vi "plots2DAnd3D.vi"() -> ()   [LabVIEW 2014]
uses:
  <vilib>/Math Plots/2D Math Plots/2D Error Bar/2D Error Bar XCtrl/2D Error Bar.xctl
  <vilib>/Math Plots/3D Math Plots/3D Contour/3D Contour XCtrl/3D Contour.xctl
  <vilib>/Math Plots/2D Math Plots/2D Error Bar/2D Error Bar Datatype/Public/Plot Helper (Percentage).vi
  <vilib>/Math Plots/3D Math Plots/3D Contour/3D Contour Datatype/Public/Plot Helper (Matrix).vi
  <vilib>/Math Plots/2D Math Plots/2D Error Bar/2D Error Bar Datatype/2D Error Bar Datatype.lvclass
  <vilib>/Math Plots/3D Math Plots/3D Contour/3D Contour Datatype/3D Contour Datatype.lvclass
panel:
  out "Contour Plotting Error":errorcluster
  in  "Frequency":dbl(knob) scale=0.0..100.0
  out "3D Contour":refnum<class "3D Plot Datatype.lvclass">[](xcontrol)
  in  "Lower Error (%)":dbl(slide) scale=0.0..10.0
  in  "Upper Error (%)":dbl(slide) scale=0.0..10.0
  out "Errorbar Plotting Error":errorcluster
  in  "Number of Points":i32(knob) scale=0.0..200.0
  out "Error Bar Plot":refnum<class "2D Plot Datatype.lvclass">[](xcontrol) caption="2D Error Bar"
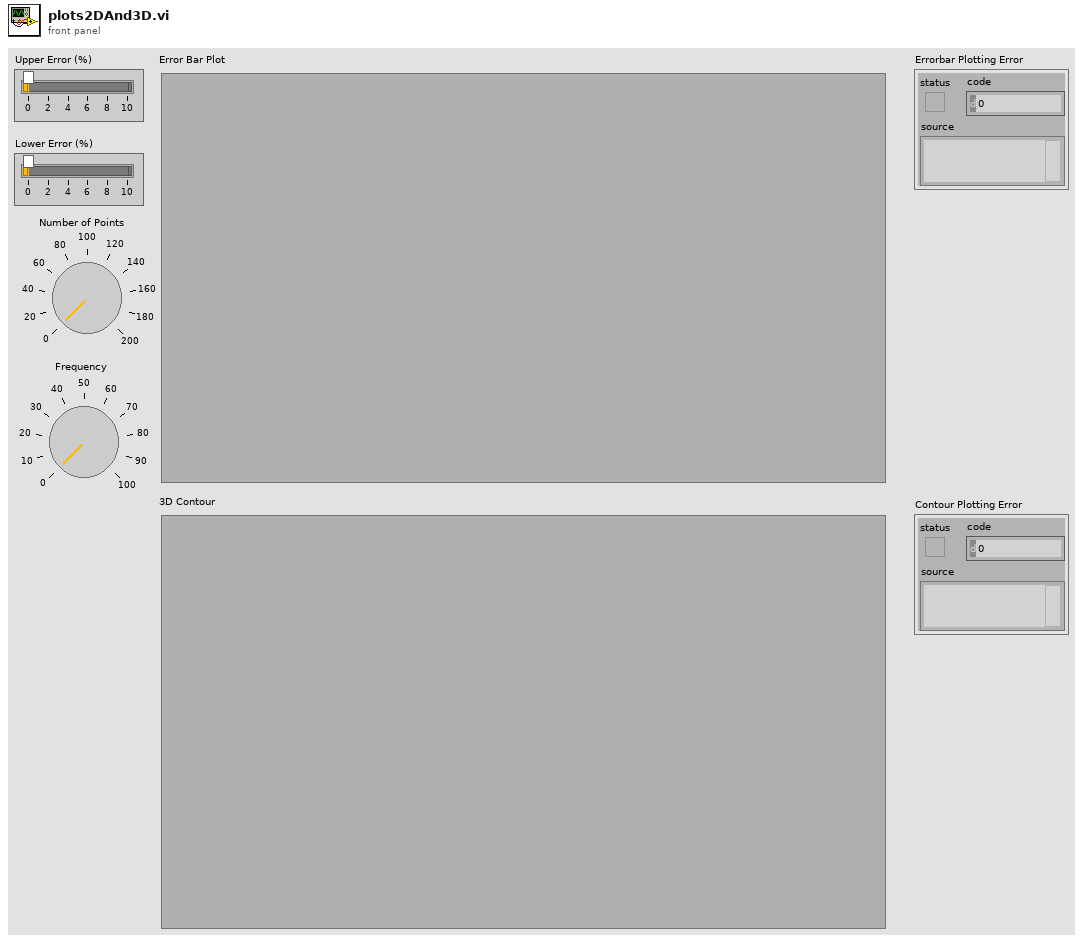
[diagram p1: front panel]
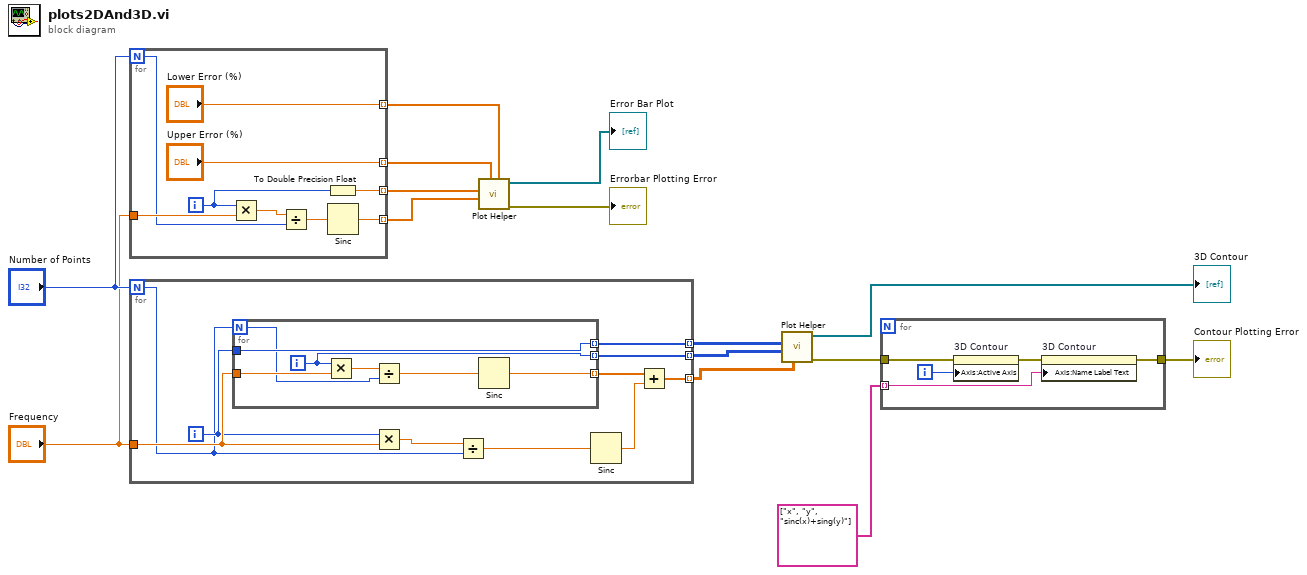
[diagram p0: block diagram]
diagram:
  n1 = for {
    N: "Number of Points" -> [w16]
    tunnel: [w24] -> w14 mode=indexing
    tunnel: [w23] -> w13 mode=indexing
    tunnel: ["Lower Error (%)"] -> w11 mode=indexing
    tunnel: ["Upper Error (%)"] -> w10 mode=indexing
    tunnel: "Frequency" -> [w19]
    i -> [w20]
    n2 = Multiply(x=w20, y=w19) -> (x*y=w17:dbl)
    n3 = Divide(x=w17, y=w16) -> (x/y=w18:dbl)
    n4 = To Double Precision Float(number=w20) -> (double precision float=w23:dbl)
    n5 = Sinc(1:w18) -> (0:w24:dbl)
  }
  n6 = for {
    N: "Number of Points" -> [w25]
    tunnel: [w32] -> w7 mode=indexing
    tunnel: "Frequency" -> [w31]
    tunnel: [w29] -> w5 mode=indexing
    tunnel: [w28] -> w4 mode=indexing
    i -> [w30]
    n7 = for {
      N: w25 -> [w35]
      tunnel: [w41] -> w33 mode=indexing
      tunnel: w31 -> [w39]
      tunnel: [w38] -> w29 mode=indexing
      tunnel: w30 -> [w38]
      tunnel: [w37] -> w28 mode=indexing
      i -> [w37]
      n8 = Multiply(x=w37, y=w39) -> (x*y=w40:dbl)
      n9 = Divide(x=w40, y=w35) -> (x/y=w36:dbl)
      n10 = Sinc(1:w36) -> (0:w41:dbl)
    }
    n11 = Multiply(x=w30, y=w31) -> (x*y=w27:dbl)
    n12 = Divide(x=w27, y=w25) -> (x/y=w26:dbl)
    n13 = Sinc(1:w26) -> (0:w34:dbl)
    n14 = Add(x=w33, y=w34) -> (x+y=w32:dbl[])
  }
  n15 = call-poly <vilib>:"Plot Helper.vi"("error b percentage"=w11, "error a percentage"=w10, "y vector"=w14, "x vector"=w13) -> ("error out"=→"Errorbar Plotting Error":errorcluster, "2D Plot Class Obj Array out"=→"Error Bar Plot":refnum<class "2D Plot Datatype.lvclass">[])  [unwired: 2 in, 4 out]
  n16 = call-poly <vilib>:"Plot Helper.vi"("z matrix"=w7, "y matrix"=w4, "x matrix"=w5) -> ("error out"=w3:errorcluster, "3D Plot lvclass Array out"=→"3D Contour":refnum<class "3D Plot Datatype.lvclass">[])  [unwired: 3 in, 4 out]
  n17 = for {
    tunnel: w3 -> [w45]
    tunnel: [w43] -> w2
    tunnel: string[] ["x", "y", "sinc(x)+sing(y)"] -> [w42] mode=indexing
    i -> [w46]
    n18 = property on="3D Contour" class="3D Contour (strict)"(error in=w45, "Axis:Active Axis"=w46) -> (error out=w44:errorcluster)  [unwired: 1 in, 1 out]
    n19 = property on="3D Contour" class="3D Contour (strict)"(error in=w44, "Axis:Name Label Text"=w42) -> (error out=w43:errorcluster)  [unwired: 1 in, 1 out]
  }
  "Contour Plotting Error" <- w2
